vi "updateTriggerQueue.vi"(8 "error in (no error)":errorcluster, 11 "Trigger queue in":refnum<queue>) -> (0 "error out":errorcluster, 2 "timed out?":bool, 3 "Trigger message":T3)   [LabVIEW 2017]
uses:
  Trigger message.ctl
panel:
  in  "Trigger list":T1(array[cluster])
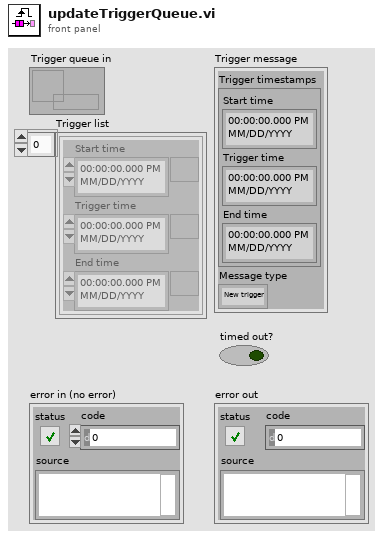
[diagram p1: front panel]
types:
  T1 = cluster{"Start time":timestamp, "Trigger time":timestamp, "End time":timestamp}[]
  T2 = typedef "Trigger message.ctl" = enum16{"New trigger", "Updated trigger"}
  T3 = cluster{"Trigger timestamps":cluster{"Start time":timestamp, "Trigger time":timestamp, "End time":timestamp}, "Message type":T2}
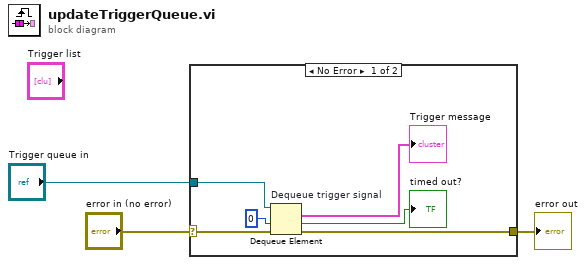
[diagram p0: block diagram]
diagram:
  n1 = case shown="No Error" "error in (no error)" {
    selector: "error in (no error)" -> [w5 w10]
    tunnel: [w8 w10] -> w3
    tunnel: "Trigger queue in" -> [w4 _]
    frame No Error {
      n2 = Dequeue Element "Dequeue trigger signal"(queue=w4, timeout in ms (-1)=0, error in (no error)=w5) -> (element=→"Trigger message":T3, timed out?=→"timed out?":bool, error out=w8:errorcluster)  [unwired: 1 out]
    }
    frame Error {
    }
  }
  "error out" <- w3
